vi "process.vi"(8 "error in (no error)":errorcluster, 11 "ClassPrivateData in":refnum<class "ClassPrivateData.lvclass">) -> (0 "error out":errorcluster, 3 "ClassPrivateData out":refnum<class "ClassPrivateData.lvclass">)   [LabVIEW 2016, in "ClassPrivateData.lvclass"]
uses:
  ClassPrivateData.lvclass
  C:/LSST_TS/SystemSW/ct_tools/ProjectItem/ProjectItem.lvclass
  Dependency/Dependency.lvclass
  ProjectItem/ProjectItem.lvclass/ProjectItem.ctl
  Dependency/Dependency.lvclass/Dependency.ctl
  ProjectItem/ProjectItem.lvclass
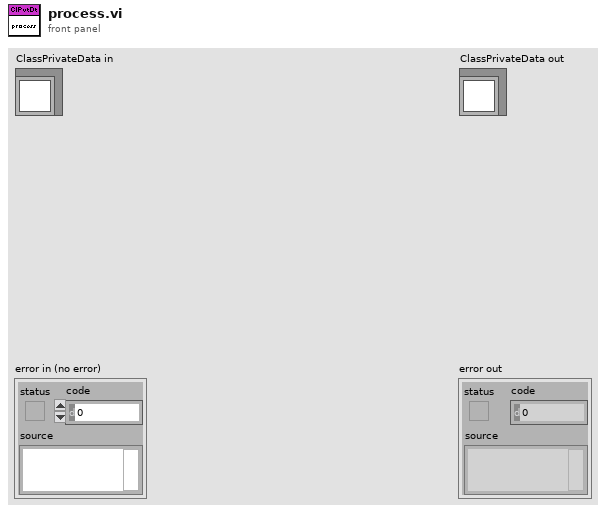
[diagram p1: front panel]
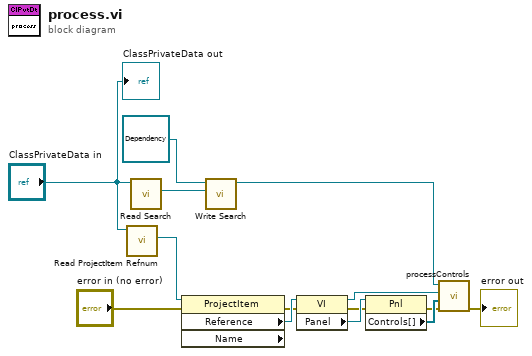
[diagram p0: block diagram]
diagram:
  n1 = call "Read ProjectItem Refnum.vi"("ProjectItem in"="ClassPrivateData in") -> ("ProjectItem Refnum"=w9:refnum<vi>)  [unwired: 9 in, 1 out]
  n2 = call "Read Search.vi"("ProjectItem in"="ClassPrivateData in") -> ("Search"=w7:refnum<class "Search.lvclass">)  [unwired: 9 in, 1 out]
  n3 = property class="ProjectItem" props=["Reference", "Name"](reference=w9, error in="error in (no error)") -> (error out=w2:errorcluster, "Reference"=w8:refnum<vi>)  [unwired: 2 out]
  n4 = call "Write Search.vi"("Search"=w7, "Dependency in"=refnum<class "Dependency.lvclass"> refnum ("Dependency.lvclass")) -> ("Dependency out"=w6:refnum<class "Dependency.lvclass">)  [unwired: 9 in]
  n5 = property class="VI"(reference=w8, error in=w2) -> (reference out=w5:refnum<vi>, error out=w13:errorcluster, "Panel"=w14:refnum<vi>)
  n6 = property class="Pnl"(reference=w14, error in=w13) -> (error out=w11:errorcluster, "Controls[]"=w12:refnum<vi>[])  [unwired: 1 out]
  n7 = call "processControls.vi"("error in (no error)"=w11, "Controls[]"=w12, "Calling VI Reference i"=w5, "Dependency in"=w6) -> ("error out"=→"error out":errorcluster)  [unwired: 5 in, 2 out]
  "ClassPrivateData out" <- "ClassPrivateData in"
